vi "Write URL.vi"(8 "error in (no error)":errorcluster, 10 "uri":string, 11 "WebView2 Control in":refnum<class "WebView2 Control.lvclass">) -> (0 "error out":errorcluster, 3 "WebView2 Control out":refnum<class "WebView2 Control.lvclass">)   [LabVIEW 2020, in "WebView2.lvlib" / "WebView2 Control.lvclass"]
uses:
  WebView2 Control.lvclass
  WebView2 Control.lvclass/WebView2 Control.ctl
  C:/Users/Simon/Documents/GitHub/LV-WebView2/Source/Libs/Microsoft.Web.WebView2.Core.dll
  Libs/Microsoft.Web.WebView2.Core.dll
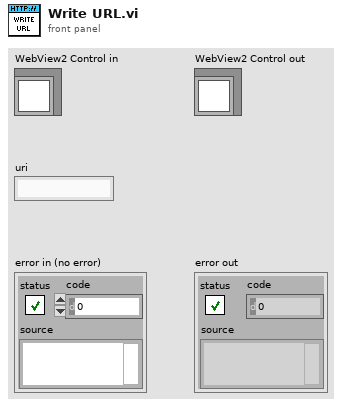
[diagram p1: front panel]
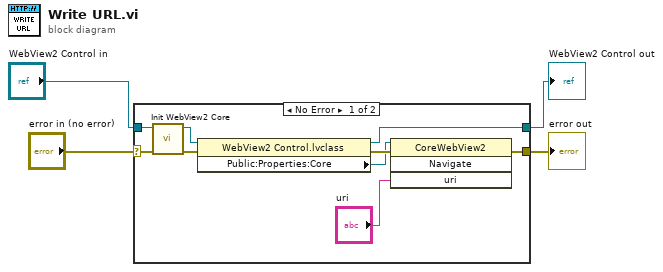
[diagram p0: block diagram]
diagram:
  n1 = case shown="No Error" "error in (no error)" {
    selector: "error in (no error)" -> [w12 w15]
    tunnel: [w6 w15] -> w3
    tunnel: [w5 w14] -> w1
    tunnel: "WebView2 Control in" -> [w13 w14]
    frame No Error {
      n2 = call "Init WebView2 Core.vi"("error in (no error)"=w12, "WebView2"=w13) -> ("error out"=w11:errorcluster, "WebView2.lvlib:WebView2 Control.lvclass"=w9:refnum<class "WebView2 Control.lvclass">)  [unwired: 8 in]
      n3 = property class="WebView2 Control.lvclass"(reference=w9, error in=w11) -> (reference out=w5:refnum<class "WebView2 Control.lvclass">, error out=w10:errorcluster, "Public:Properties:Core"=w8:refnum<k24>)
      n4 = invoke class="CoreWebView2" method="Navigate"(reference=w8, error in=w10, "uri"="uri") -> (error out=w6:errorcluster)  [unwired: 1 in, 3 out]
    }
    frame Error {
    }
  }
  "error out" <- w3
  "WebView2 Control out" <- w1
